vi "Create.vi"(8 "error in (no error)":errorcluster) -> (0 "error out":errorcluster, 3 "Main out":refnum<class "Main.lvclass">)   [LabVIEW 2020, in "Main.lvclass"]
uses:
  Main.lvclass
  Debugger/Debugger.lvclass
  C:/Users/anton/Documents/GitHub/triarc-debugger/source/Process/Debug Process.lvclass
  C:/Users/anton/Documents/GitHub/triarc-debugger/source/Debug Data Event/Debug Data Listener.lvclass
  Debug Message Receiver/Debug Message Receiver.lvclass
  List Seen Messages View Model/List Messages View Model.lvclass
  C:/Users/anton/Documents/GitHub/triarc-debugger/source/List Box View Model_/List Box View Model.lvclass
  List View/List Box View.lvclass
  C:/Users/anton/Documents/GitHub/triarc-debugger/source/Debug View/Debug View.lvclass
  List Seen Processes View Model/List Processes View Model.lvclass
  Process/Debug Process.lvclass/Debug Process.ctl
  Debug Message Receiver/Debug Message Receiver.lvclass/Debug Message Receiver.ctl
  List View/List Box View.lvclass/List Box View.ctl
  Process/Public/Lifecycle/Get Lifecycle State.vi
  Process/Protected/Messaging/Enqueue Message.vi
  <vilib>/Utility/error.llb/Clear Errors.vi
  <vilib>/Utility/error.llb/Error Cluster From Error Code.vi
  Process/Debug Process.lvclass
  Debug View/Debug View.lvclass
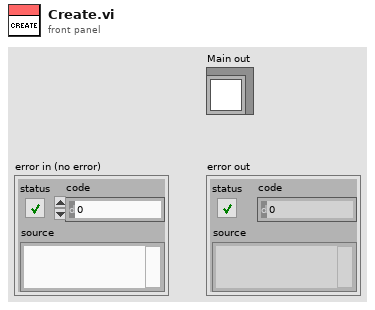
[diagram p1: front panel]
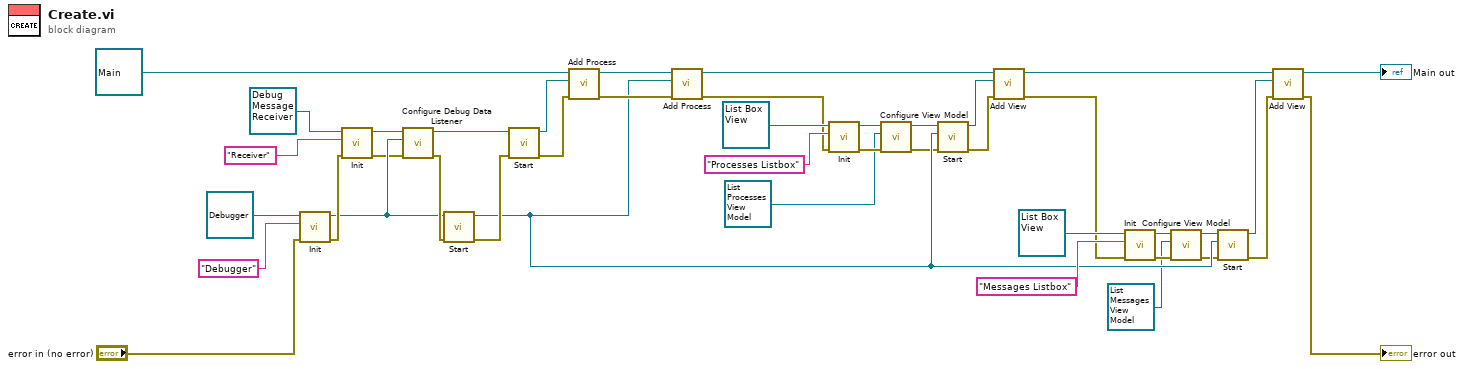
[diagram p0: block diagram]
diagram:
  n1 = call-dynamic "Init.vi"("error in (no error)"="error in (no error)", "Name"="Debugger", "Process In"=refnum<class "Debugger.lvclass"> refnum ("Debugger.lvclass")) -> ("error out"=w37:errorcluster, "Process Out"=w36:refnum<class "Debugger.lvclass">)  [unwired: 7 in]
  n2 = call-dynamic "Init.vi"("error in (no error)"=w37, "Name"="Receiver", "Process In"=refnum<class "Debug Message Receiver.lvclass"> refnum ("Debug Message Receiver.lvclass")) -> ("error out"=w31:errorcluster, "Process Out"=w34:refnum<class "Debug Message Receiver.lvclass">)  [unwired: 7 in]
  n3 = call "Configure Debug Data Listener.vi"("error in (no error)"=w31, "Debug Data Listener"=w36, "Debug Message Receiver In"=w34) -> ("error out"=w39:errorcluster, "Debug Message Receiver Out"=w32:refnum<class "Debug Message Receiver.lvclass">)  [unwired: 7 in]
  n4 = call "Start.vi"("error in (no error)"=w39, "Process In"=w36) -> ("error out"=w40:errorcluster, "Process Out"=w10:refnum<class "Debugger.lvclass">)  [unwired: 7 in, 1 out]
  n5 = call "Start.vi"("error in (no error)"=w40, "Process In"=w32) -> ("error out"=w25:errorcluster, "Process Out"=w27:refnum<class "Debug Message Receiver.lvclass">)  [unwired: 7 in, 1 out]
  n6 = call "Add Process.vi"("error in (no error)"=w25, "Debug Process"=w27, "Main In"=refnum<class "Main.lvclass"> refnum ("Main in")) -> ("error out"=w26:errorcluster, "Main Out"=w30:refnum<class "Main.lvclass">)  [unwired: 7 in]
  n7 = call "Add Process.vi"("error in (no error)"=w26, "Debug Process"=w10, "Main In"=w30) -> ("error out"=w15:errorcluster, "Main Out"=w28:refnum<class "Main.lvclass">)  [unwired: 7 in]
  n8 = call-dynamic "Init.vi"("error in (no error)"=w15, "Name"="Processes Listbox", "Debug View In"=refnum<class "List Box View.lvclass"> refnum ("List Box View.lvclass")) -> ("error out"=w7:errorcluster, "Debug View Out"=w9:refnum<class "List Box View.lvclass">)  [unwired: 7 in]
  n9 = call "Configure View Model.vi"("error in (no error)"=w7, "List Box View Model"=refnum<class "List Processes View Model.lvclass"> refnum ("List Processes View Model.lvclass"), "List Box View In"=w9) -> ("error out"=w6:errorcluster, "List Box View Out"=w8:refnum<class "List Box View.lvclass">)  [unwired: 7 in]
  n10 = call "Start.vi"("error in (no error)"=w6, "Context"=w10, "Debug View In"=w8) -> ("error out"=w16:errorcluster, "Debug View Out"=w17:refnum<class "List Box View.lvclass">)  [unwired: 7 in]
  n11 = call "Add View.vi"("error in (no error)"=w16, "Debug Process"=w17, "Main In"=w28) -> ("error out"=w14:errorcluster, "Main Out"=w19:refnum<class "Main.lvclass">)  [unwired: 7 in]
  n12 = call-dynamic "Init.vi"("error in (no error)"=w14, "Name"="Messages Listbox", "Debug View In"=refnum<class "List Box View.lvclass"> refnum ("List Box View.lvclass")) -> ("error out"=w23:errorcluster, "Debug View Out"=w3:refnum<class "List Box View.lvclass">)  [unwired: 7 in]
  n13 = call "Configure View Model.vi"("error in (no error)"=w23, "List Box View Model"=refnum<class "List Messages View Model.lvclass"> refnum ("List Messages View Model.lvclass"), "List Box View In"=w3) -> ("error out"=w4:errorcluster, "List Box View Out"=w2:refnum<class "List Box View.lvclass">)  [unwired: 7 in]
  n14 = call "Start.vi"("error in (no error)"=w4, "Context"=w10, "Debug View In"=w2) -> ("error out"=w12:errorcluster, "Debug View Out"=w11:refnum<class "List Box View.lvclass">)  [unwired: 7 in]
  n15 = call "Add View.vi"("error in (no error)"=w12, "Debug Process"=w11, "Main In"=w19) -> ("error out"=→"error out":errorcluster, "Main Out"=→"Main out":refnum<class "Main.lvclass">)  [unwired: 7 in]
